vi "Upload.vi"(8 "INO":path, 9 "CLI":path, 11 "Selector":string(combo)) -> (3 "Comando_Upload":string)   [LabVIEW 2025]
doc: "Crea el comando para subir el firmware a partir del puerto COM seleccionado"
uses:
  <vilib>/Utility/error.llb/Trim Whitespace One-Sided.vi
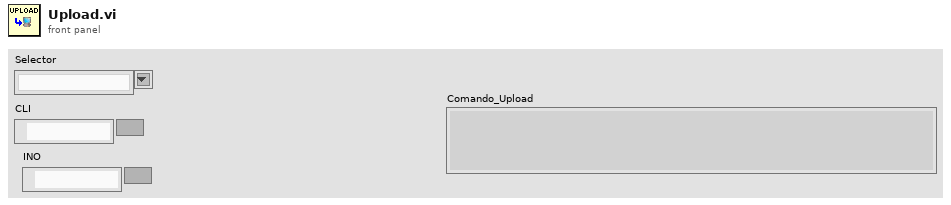
[diagram p1: front panel]
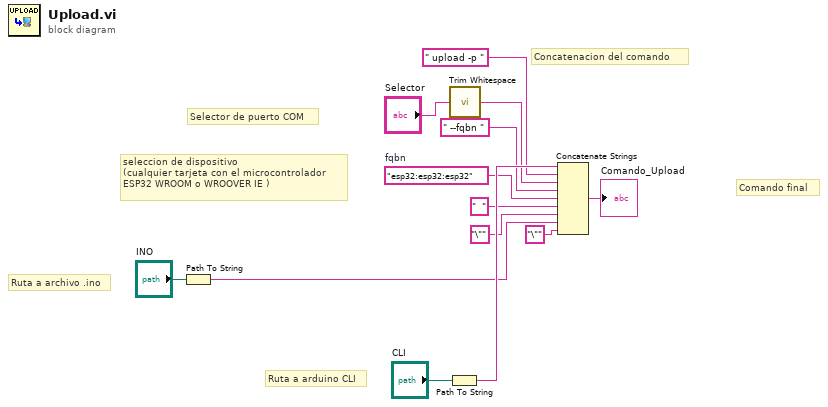
[diagram p0: block diagram]
diagram:
  w7 = "esp32:esp32:esp32"  # fqbn
  # "Selector de puerto COM"
  # "Comando final"
  # "Concatenacion del comando"
  # "seleccion de dispositivo\n(cualquier tarjeta con el microcontrolador \nESP32 WROOM o WROOVER IE )"
  # "Ruta a archivo .ino"
  # "Ruta a arduino CLI"
  n1 = Path To String(path="INO") -> (string=w3:string)
  n2 = Path To String(path="CLI") -> (string=w12:string)
  n3 = call <vilib>:"Trim Whitespace.vi"("string"="Selector") -> ("trimmed string"=w10:string)  [unwired: 1 in]
  n4 = Concatenate Strings(w12, " upload -p " ("string"), w10, " --fqbn " ("string"), w7, "  " ("string"), "\"" ("string"), w3, "\"" ("string")) -> (→"Comando_Upload":string)
